vi "SetupApplication.vi"(8 "error in (no error)":errorcluster, 11 "EVE reference in":refnum<data-value>) -> (0 "error out":errorcluster, 3 "EVE reference out":refnum<data-value>)   [LabVIEW 2013]
uses:
  Class/EVE/EVE.lvclass
  050 - CONFIG/00 - ApplicationConfig/Ctrls/EnumFgvConfigCommand.ctl
  080 - TOOLS/Traduction/Dictionnary/EnumCommandDictionnaire.ctl
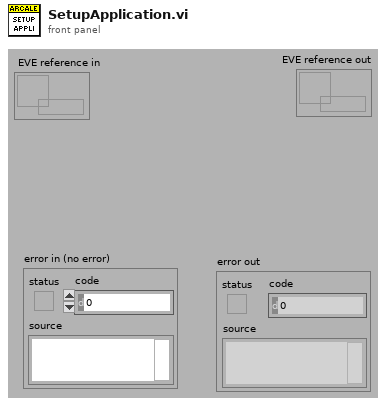
[diagram p1: front panel]
types:
  T1 = typedef "EnumCommandDictionnaire.ctl" = enum16{"Load", "Translate", "Save", "GetDico", "Set : A traduire = Vrai", "Set : A Traduire = Faux", "SetDico"}
  T2 = typedef "EnumFgvConfigCommand.ctl" = enum16{"Load", "Get", "Set", "Save To Disk"}
  T3 = typedef "ApplicationConfig.ctl" = cluster{"Data Path":path, "MessageHandlerConfig":T4, "Simulation":bool, "Dictionnary":string}
  T4 = typedef "MessageHandlerConfig.ctl" = cluster{"Max log files":u32, "Max messages per file":u32}
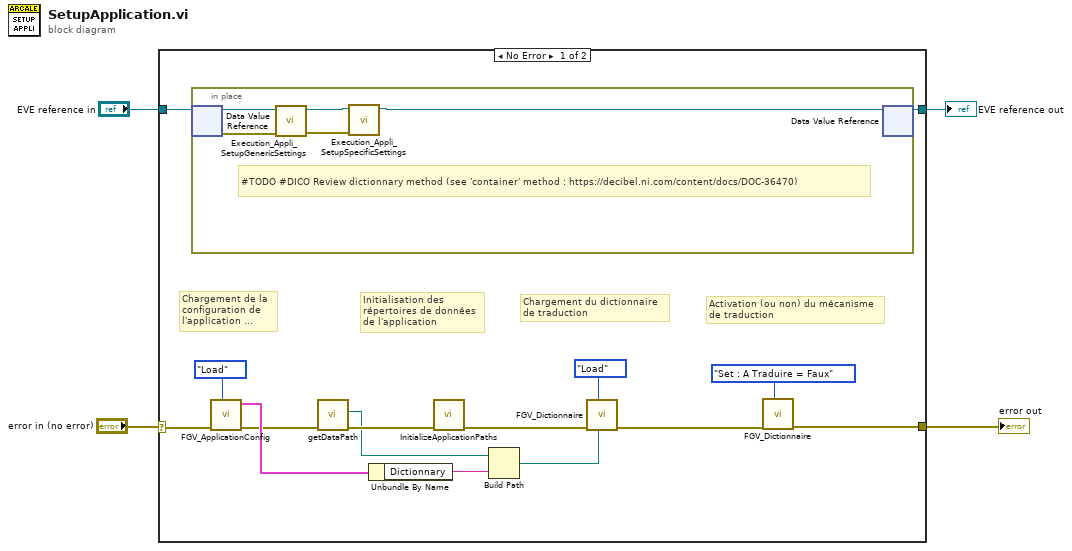
[diagram p0: block diagram]
diagram:
  n1 = case shown="No Error" "error in (no error)" {
    selector: "error in (no error)" -> [w18 w26]
    tunnel: [w13 w26] -> w3
    tunnel: "EVE reference in" -> [w6 w25]
    tunnel: [w5 w25] -> w1
    frame No Error {
      # "Activation (ou non) du mécanisme\nde traduction"
      # "Chargement du dictionnaire\nde traduction"
      # "Initialisation des\nrépertoires de données\nde l'application"
      # "Chargement de la \nconfiguration de \nl'application ..."
      n2 = in-place {
        # "#TODO #DICO Review dictionnary method (see 'container' method : https://decibel.ni.com/content/docs/DOC-36470)"
        n3 = in-place-dvr #1(w6) -> (w24:refnum<class "EVE.lvclass">, w23:errorcluster)
        n4 = call-dynamic "Execution_Appli_SetupGenericSettings.vi"("error in"=w23, "EVE in"=w24) -> ("error out"=w20:errorcluster, "EVE out"=w22:refnum<class "EVE.lvclass">)  [unwired: 8 in]
        n5 = call-dynamic "Execution_Appli_SetupSpecificSettings.vi"("error in"=w20, "EVE in"=w22) -> ("EVE out"=w21:refnum<class "EVE.lvclass">)  [unwired: 8 in, 1 out]
        n6 = in-place-dvr #1(w21) -> (w5:refnum<data-value>)  [unwired: 1 out]
      }
      n7 = call "FGV_ApplicationConfig.vi"("Command"=EnumFgvConfigCommand."Load", "error in (no error)"=w18) -> ("error out"=w9:errorcluster, "ApplicationConfigOut"=w12:T3)  [unwired: 8 in]
      n8 = call "getDataPath.vi"("error in (no error)"=w9) -> ("error out"=w8:errorcluster, "DataPath"=w7:path)  [unwired: 9 in]
      n9 = Unbundle By Name(w12) -> ("Dictionnary"=w11:string)
      n10 = call "InitializeApplicationPaths.vi"("error in (no error)"=w8) -> ("error out"=w17:errorcluster)  [unwired: 10 in]
      n11 = Build Path(base path=w7, name or relative path=w11) -> (appended path=w10:path)
      n12 = call "FGV_Dictionnaire.vi"("FichierDictionnaire"=w10, "Command"=EnumCommandDictionnaire."Load", "error in (no error)"=w17) -> ("error out"=w15:errorcluster)  [unwired: 6 in, 2 out]
      n13 = call "FGV_Dictionnaire.vi"("Command"=EnumCommandDictionnaire."Set : A Traduire = Faux", "error in (no error)"=w15) -> ("error out"=w13:errorcluster)  [unwired: 7 in, 2 out]
    }
    frame Error {
    }
  }
  "error out" <- w3
  "EVE reference out" <- w1
